vi "TCP Engine Read configuration data.vi"(6 "AI":path, 9 "Serial":path, 10 "DI":path, 11 "DO":path) -> (1 "Async data":T8 {"Interface Data"."Data"."Minor Frame Count" min=5 max=8 step=1}, 2 "DO data":T1, 3 "DI data":T1, 4 "AI data":T4={"Interface"="AIO", "Interface Data"={"Command"="Configure", "SubCmd"="AO", "Data"=[], "Timing"={"samples per channel"=1000, "sample mode"=10178, "Sampling Rate"=1000.0}}} {"Interface Data"."Timing"."sample mode" items=["Finite Samples"=10178, "Continuous Samples"=10123, "Hardware Timed Single Point"=12522]})   [LabVIEW 2024]
uses:
  Digital Output/Controls/DIO Configuration cluster.ctl
  Digital Output/Controls/DIO Interface Data.ctl
  Digital Output/SubVIs/Digital Dynamic Cluster.ctl
  Host/Async JSON Cluster.ctl
  Host/Async Interface Data Cluster.ctl
  Async Serial/Controls/Async Serial Configuration Cluster.ctl
  Async Serial/Controls/Async Frame Info Cluster.ctl
  Async Serial/Controls/Async Message Info Cluster.ctl
  Analog Output/Controls/AO JSON Data Cluster.ctl
  Analog Output/Controls/AO Interface Data Cluster.ctl
  Analog Output/Controls/AO Channel Configuration Cluster.ctl
  Analog Output/Controls/AO Timing Cluster.ctl
  <vilib>/Utility/config.llb/NI_LVConfig.lvlib
  <userlib>/_OpenG.lib/variantconfig/variantconfig.llb/openg_variant_configuration_file.lvlib
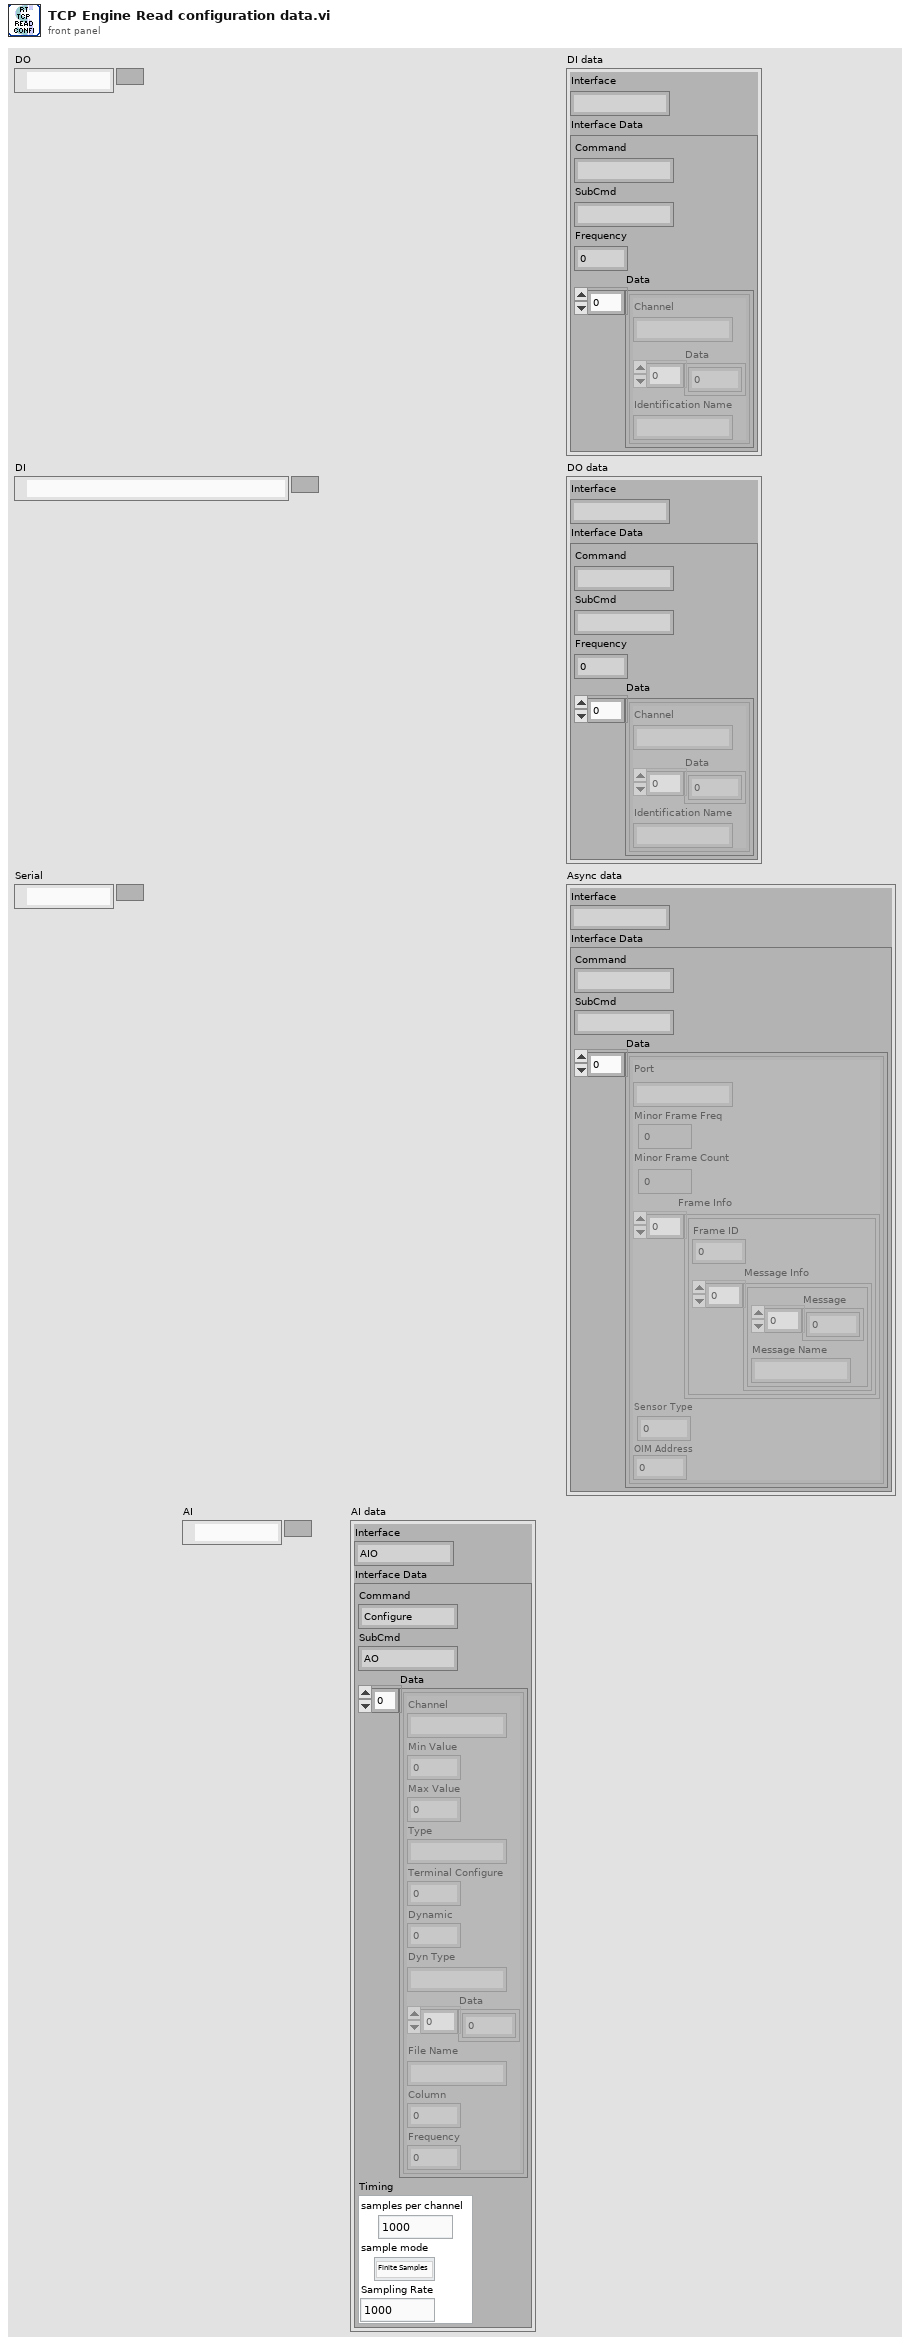
[diagram p1: front panel]
types:
  T1 = typedef "DIO Configuration cluster.ctl" = cluster{"Interface":string, "Interface Data":T2}
  T2 = typedef "DIO Interface Data.ctl" = cluster{"Command":string, "SubCmd":string, "Frequency":u16, "Data":T3[]}
  T3 = typedef "Digital Dynamic Cluster.ctl" = cluster{"Channel":string, "Data":u8[], "Identification Name":string}
  T4 = typedef "AO JSON Data Cluster.ctl" = cluster{"Interface":string, "Interface Data":T5}
  T5 = typedef "AO Interface Data Cluster.ctl" = cluster{"Command":string, "SubCmd":string, "Data":T6[], "Timing":T7}
  T6 = typedef "AO Channel Configuration Cluster.ctl" = cluster{"Channel":string, "Min Value":dbl, "Max Value":dbl, "Type":string, "Terminal Configure":u16, "Dynamic":u8, "Dyn Type":string, "Data":dbl[], "File Name":string, "Column":i32, "Frequency":dbl}
  T7 = typedef "AO Timing Cluster.ctl" = cluster{"samples per channel":i32, "sample mode":i32, "Sampling Rate":dbl}
  T8 = typedef "Async JSON Cluster.ctl" = cluster{"Interface":string, "Interface Data":T9}
  T9 = typedef "Async Interface Data Cluster.ctl" = cluster{"Command":string, "SubCmd":string, "Data":T10[]}
  T10 = typedef "Async Serial Configuration Cluster.ctl" = cluster{"Port":string, "Minor Frame Freq":u16, "Minor Frame Count":u16, "Frame Info":T11[], "Sensor Type":u16, "OIM Address":u16}
  T11 = typedef "Async Frame Info Cluster.ctl" = cluster{"Frame ID":u16, "Message Info":T12[]}
  T12 = typedef "Async Message Info Cluster.ctl" = cluster{"Message":u8[], "Message Name":string}
  T13 = typedef "NI_LVConfig.lvlib/Config Data RefNum.ctl" = refnum<k1>
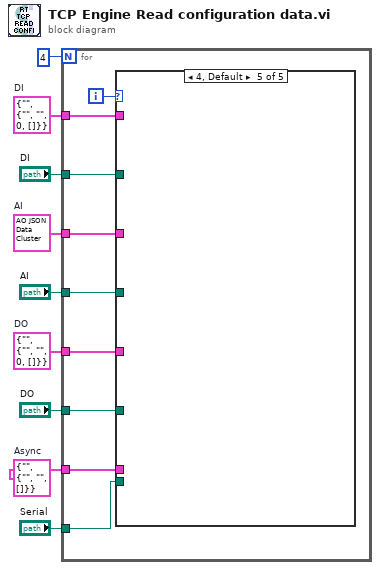
[diagram p0: block diagram]
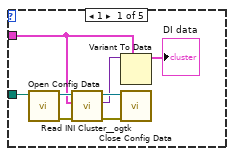
[diagram p2: hidden frame]
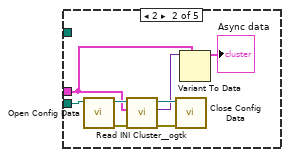
[diagram p3: hidden frame]
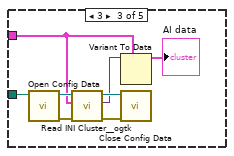
[diagram p4: hidden frame]
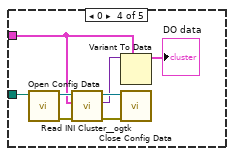
[diagram p5: hidden frame]
diagram:
  w7 = T8 {"Interface"="", "Interface Data"={"Command"="", "SubCmd"="", "Data"=[]}}  # Async
  w8 = T4 {"Interface"="AIO", "Interface Data"={"Command"="Configure", "SubCmd"="AO", "Data"=[], "Timing"={"samples per channel"=1000, "sample mode"=10178, "Sampling Rate"=1000.0}}}  # AI
  w3 = T1 {"Interface"="", "Interface Data"={"Command"="", "SubCmd"="", "Frequency"=0, "Data"=[]}}  # DO
  w4 = T1 {"Interface"="", "Interface Data"={"Command"="", "SubCmd"="", "Frequency"=0, "Data"=[]}}  # DI
  n1 = for {
    N: 4 -> [_]
    tunnel: "DO" -> [w17]
    tunnel: w3 -> [w16]
    tunnel: w4 -> [w15]
    tunnel: "DI" -> [w14]
    tunnel: "Serial" -> [w13]
    tunnel: w7 -> [w12]
    tunnel: w8 -> [w11]
    tunnel: "AI" -> [w10]
    i -> [w18]
    n2 = case shown="4, Default" w18 {
      tunnel: w17 -> [_ _ _ w46 _]
      tunnel: w16 -> [_ _ _ w43 _]
      tunnel: w15 -> [w19 _ _ _ _]
      tunnel: w14 -> [w22 _ _ _ _]
      tunnel: w13 -> [_ w30 _ _ _]
      tunnel: w12 -> [_ w28 _ _ _]
      tunnel: w11 -> [_ _ w36 _ _]
      tunnel: w10 -> [_ _ w38 _ _]
      frame 1 {
        n3 = call <vilib>:"Open Config Data.vi"("configuration file path"=w22) -> ("error out"=w24:errorcluster, "refnum"=w26:T13)  [unwired: 8 in, 1 out]
        n4 = call <userlib>:"Read INI Cluster__ogtk.vi"("error in (no error)"=w24, "INI Fomatted Cluster Type"=w19, "refnum"=w26) -> ("error out"=w23:errorcluster, "INI Fomatted Cluster"=w21:variant, "dup refnum"=w25:T13)  [unwired: 4 in, 2 out]
        n5 = Variant To Data(type=w19, Variant=w21) -> (data=→"DI data":T1)  [unwired: 1 in, 1 out]
        n6 = call <vilib>:"Close Config Data.vi"("error in (no error)"=w23, "refnum"=w25) -> ()  [unwired: 8 in, 2 out]
      }
      frame 2 {
        n7 = call <vilib>:"Open Config Data.vi"("configuration file path"=w30) -> ("error out"=w32:errorcluster, "refnum"=w34:T13)  [unwired: 8 in, 1 out]
        n8 = call <userlib>:"Read INI Cluster__ogtk.vi"("error in (no error)"=w32, "INI Fomatted Cluster Type"=w28, "refnum"=w34) -> ("error out"=w31:errorcluster, "INI Fomatted Cluster"=w29:variant, "dup refnum"=w33:T13)  [unwired: 4 in, 2 out]
        n9 = call <vilib>:"Close Config Data.vi"("error in (no error)"=w31, "refnum"=w33) -> ()  [unwired: 8 in, 2 out]
        n10 = Variant To Data(type=w28, Variant=w29) -> (data=→"Async data":T8)  [unwired: 1 in, 1 out]
      }
      frame 3 {
        n11 = call <vilib>:"Open Config Data.vi"("configuration file path"=w38) -> ("error out"=w40:errorcluster, "refnum"=w42:T13)  [unwired: 8 in, 1 out]
        n12 = call <userlib>:"Read INI Cluster__ogtk.vi"("error in (no error)"=w40, "INI Fomatted Cluster Type"=w36, "refnum"=w42) -> ("error out"=w39:errorcluster, "INI Fomatted Cluster"=w37:variant, "dup refnum"=w41:T13)  [unwired: 4 in, 2 out]
        n13 = Variant To Data(type=w36, Variant=w37) -> (data=→"AI data":T4)  [unwired: 1 in, 1 out]
        n14 = call <vilib>:"Close Config Data.vi"("error in (no error)"=w39, "refnum"=w41) -> ()  [unwired: 8 in, 2 out]
      }
      frame 0 {
        n15 = call <vilib>:"Open Config Data.vi"("configuration file path"=w46) -> ("error out"=w48:errorcluster, "refnum"=w50:T13)  [unwired: 8 in, 1 out]
        n16 = call <userlib>:"Read INI Cluster__ogtk.vi"("error in (no error)"=w48, "INI Fomatted Cluster Type"=w43, "refnum"=w50) -> ("error out"=w47:errorcluster, "INI Fomatted Cluster"=w45:variant, "dup refnum"=w49:T13)  [unwired: 4 in, 2 out]
        n17 = Variant To Data(type=w43, Variant=w45) -> (data=→"DO data":T1)  [unwired: 1 in, 1 out]
        n18 = call <vilib>:"Close Config Data.vi"("error in (no error)"=w47, "refnum"=w49) -> ()  [unwired: 8 in, 2 out]
      }
      frame 4, Default {
      }
    }
  }
